vi "Remove Panel.vi"(0 "Shelf Number":string, 6 "connection information":path, 7 "System Num":u32=1 min=1 max=6) -> ()   [LabVIEW 2024]
uses:
  <vilib>/addons/database/Connection.llb/DB Tools Open Connec (Path).vi
  <vilib>/addons/database/Connection.llb/Conn Execute.vi
  <vilib>/addons/database/Recordset.llb/Rec Destroy - Connection.vi
  <vilib>/addons/database/_DB Variant To Data/Database Variant To Data.xnode
  <vilib>/addons/database/NI_Database_API.lvlib
panel:
  in  "Active Positions 2":string
  in  "Deselect All 2":bool
  in  "Select All 2":bool
  out "PreActive 2":string[](array[string])
  out "Rack 2":string
  out "Rack 1":string
  in  "13":bool
  in  "14":bool
  in  "15":bool
  in  "16":bool
  in  "21":bool
  in  "22":bool
  in  "23":bool
  in  "24":bool
  in  "29":bool
  in  "30":bool
  in  "31":bool
  in  "32":bool
  in  "10":bool
  in  "11":bool
  in  "12":bool
  in  "18":bool
  in  "19":bool
  in  "20":bool
  in  "26":bool
  in  "27":bool
  in  "28":bool
  in  "1":bool
  in  "2":bool
  in  "3":bool
  in  "4":bool
  in  "5":bool
  in  "6":bool
  in  "7":bool
  in  "8":bool
  in  "9":bool
  in  "17":bool
  in  "25":bool
  in  "Deselect All 1":bool
  out "PreActive 1":string[](array[string])
  out "System #":u32=1 min=1 max=6
  in  "Confirm":bool
  in  "Active Positions 1":string
  in  "13":bool
  in  "14":bool
  in  "15":bool
  in  "16":bool
  in  "21":bool
  in  "22":bool
  in  "23":bool
  in  "24":bool
  in  "29":bool
  in  "30":bool
  in  "31":bool
  in  "32":bool
  in  "10":bool
  in  "11":bool
  in  "12":bool
  in  "18":bool
  in  "19":bool
  in  "20":bool
  in  "26":bool
  in  "27":bool
  in  "28":bool
  in  "1":bool
  in  "2":bool
  in  "3":bool
  in  "4":bool
  in  "5":bool
  in  "6":bool
  in  "7":bool
  in  "8":bool
  in  "9":bool
  in  "17":bool
  in  "25":bool
  in  "Select All 1":bool
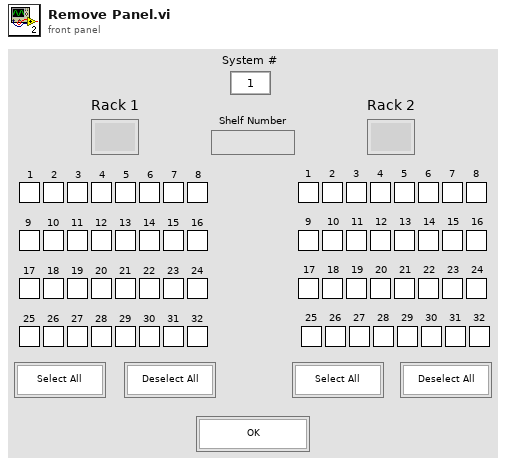
[diagram p1: front panel]
types:
  T1 = typedef "NI_Database_API.lvlib/Conn ObjectReference.ctl" = refnum<k1>
  T2 = typedef "NI_Database_API.lvlib/Rec ObjectReference.ctl" = refnum<k1>
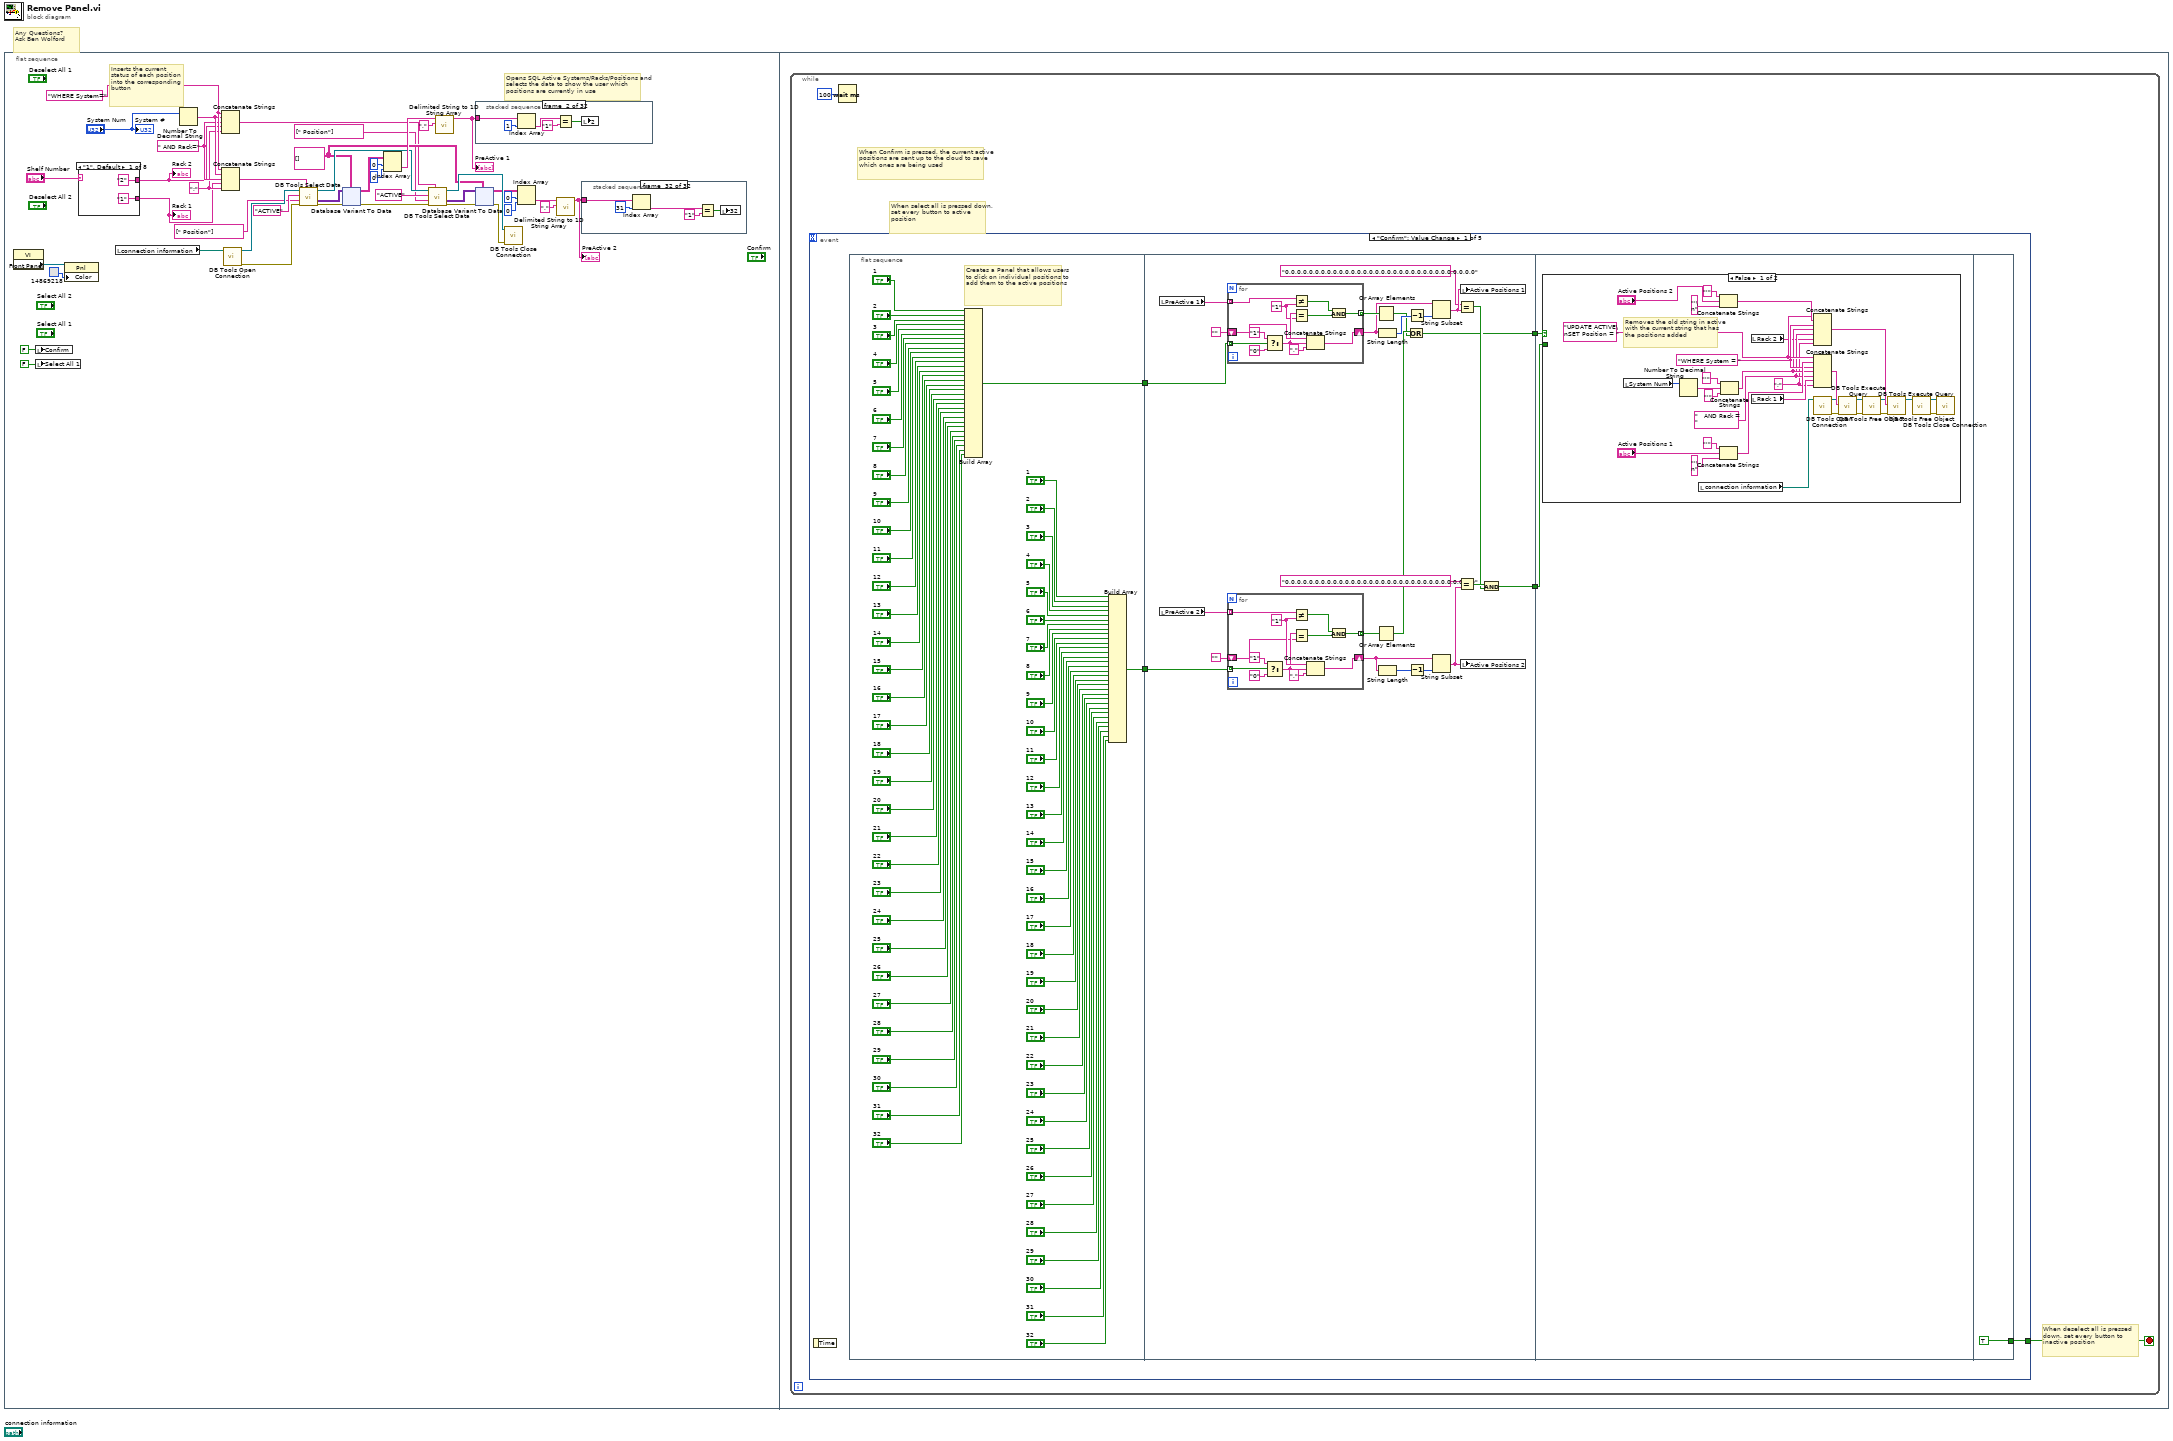
[diagram p0: block diagram]
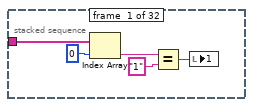
[diagram p2: hidden frame]
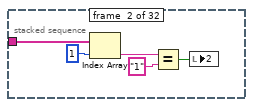
[diagram p3: hidden frame]
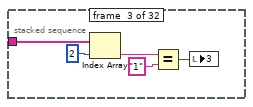
[diagram p4: hidden frame]
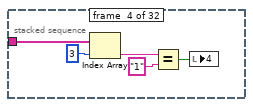
[diagram p5: hidden frame]
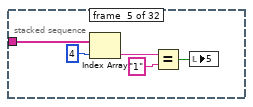
[diagram p6: hidden frame]
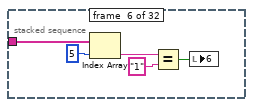
[diagram p7: hidden frame]
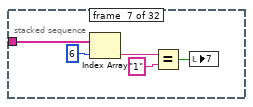
[diagram p8: hidden frame]
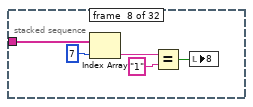
[diagram p9: hidden frame]
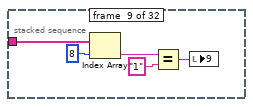
[diagram p10: hidden frame]
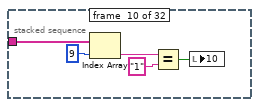
[diagram p11: hidden frame]
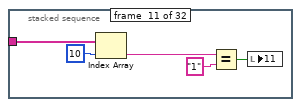
[diagram p12: hidden frame]
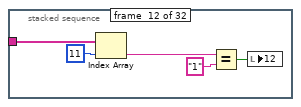
[diagram p13: hidden frame]
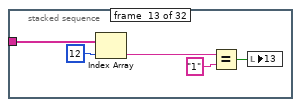
[diagram p14: hidden frame]
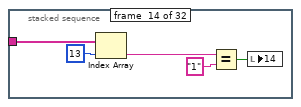
[diagram p15: hidden frame]
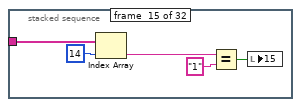
[diagram p16: hidden frame]
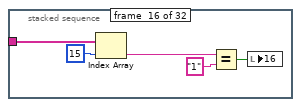
[diagram p17: hidden frame]
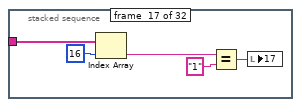
[diagram p18: hidden frame]
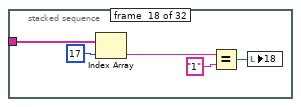
[diagram p19: hidden frame]
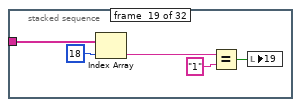
[diagram p20: hidden frame]
diagram:
  # "Any Questions? \nAsk Ben Wolford"
  n1 = flat-sequence {
    frame #0 {
      w5 = string[][] [] ("table")
      w29 = " AND Rack=" ("string")
      w28 = ";" ("string")
      w31 = "WHERE System=" ("SQL Query")
      # "Inserts the current status of each position into the corresponding button"
      # "Opens SQL Active Systems/Racks/Positions and selects the data to show the user which positions are currently in use"
      n2 = property class="VI"() -> ("Front Panel"=w34:refnum<vi>)  [unwired: 2 in, 2 out]
      n3 = local write "Confirm"(FALSE ("Confirm")) -> ()
      n4 = local write "Select All 1"(FALSE ("Select All")) -> ()
      n5 = property class="Pnl"(reference=w34, "Color"=u32 14869218) -> ()  [unwired: 1 in, 2 out]
      n6 = case shown="\"1\", Default" "Shelf Number" {
        tunnel: ["2" ("Rack 1") "4" ("Rack 1") "6" ("Rack 1") "8" ("Rack 1") "10" ("Rack 1") "12" ("Rack 1") "14" ("Rack 1") "16" ("Rack 1")] -> w26
        tunnel: ["1" ("Rack 1") "3" ("Rack 1") "5" ("Rack 1") "7" ("Rack 1") "9" ("Rack 1") "11" ("Rack 1") "13" ("Rack 1") "15" ("Rack 1")] -> w27
        frame "1", Default {
        }
        frame "2" {
        }
        frame "3" {
        }
        frame "4" {
        }
        frame "5" {
        }
        frame "6" {
        }
        frame "7" {
        }
        frame "8" {
        }
      }
      "Rack 1" <- w27
      "Rack 2" <- w26
      n7 = local read "connection information"() -> (w1:path)
      n8 = Number To Decimal String(number="System Num") -> (decimal integer string=w30:string)  [unwired: 1 in]
      n9 = Concatenate Strings(w31, w30, w29, w26, w28) -> (w4:string)
      n10 = Concatenate Strings(w31, w30, w29, w27, w28) -> (w8:string)
      n11 = call-poly <vilib>:"DB Tools Open Connection.vi"("connection information"=w1) -> ("error out"=w19:errorcluster, "connection reference"=w20:T1)  [unwired: 7 in]
      n12 = call <vilib>:"DB Tools Select Data.vi"("condition"=w8, "error in (no error)"=w19, "columns"=string[] [" Position"], "table"="ACTIVE", "connection reference"=w20) -> ("error out"=w14:errorcluster, "data"=w17:variant[][], "connection reference out"=w9:T1)  [unwired: 1 in]
      n13 = xnode "Database Variant To Data"("database variant"=w17, "error in (no error)"=w14, "type"=w5) -> ("data"=w7:string[][], "error out"=w13:errorcluster)
      n14 = Index Array(array=w7, index (row)=0, index (col)=0 ("disabled index (col)")) -> (element=w41:string)
      n15 = call <vilib>:"DB Tools Select Data.vi"("condition"=w4, "error in (no error)"=w13, "columns"=string[] [" Position"], "table"="ACTIVE", "connection reference"=w9) -> ("error out"=w12:errorcluster, "data"=w15:variant[][], "connection reference out"=w10:T1)  [unwired: 1 in]
      n16 = call <vilib>:"Delimited String to 1D String Array.vi"("delimiter"=",", "delimited string"=w41) -> ("string array"=w42:string[])  [unwired: 9 in]
      "PreActive 1" <- w42
      n17 = stacked-sequence {
        tunnel: w42 -> [w311 w313 w318 w323 w328 w333 w338 w343 w348 w353 w358 w363 w368 w373 w378 w383 w388 w393 w398 w403 w408 w413 w418 w423 w428 w433 w438 w443 w448 w453 w458 w463]
        frame #0 {
          n18 = Index Array(array=w311, index=0) -> (element=w309:string)
          n19 = Equal?(x=w309, y="1") -> (x = y?=w307:bool)
          n20 = local write "1"(w307) -> ()
        }
        frame #1 {
          n21 = Index Array(array=w313, index=1) -> (element=w315:string)
          n22 = Equal?(x=w315, y="1") -> (x = y?=w312:bool)
          n23 = local write "2"(w312) -> ()
        }
        frame #2 {
          n24 = Index Array(array=w318, index=2) -> (element=w320:string)
          n25 = Equal?(x=w320, y="1") -> (x = y?=w317:bool)
          n26 = local write "3"(w317) -> ()
        }
        frame #3 {
          n27 = Index Array(array=w323, index=3) -> (element=w325:string)
          n28 = Equal?(x=w325, y="1") -> (x = y?=w322:bool)
          n29 = local write "4"(w322) -> ()
        }
        frame #4 {
          n30 = Index Array(array=w328, index=4) -> (element=w330:string)
          n31 = Equal?(x=w330, y="1") -> (x = y?=w327:bool)
          n32 = local write "5"(w327) -> ()
        }
        frame #5 {
          n33 = Index Array(array=w333, index=5) -> (element=w335:string)
          n34 = Equal?(x=w335, y="1") -> (x = y?=w332:bool)
          n35 = local write "6"(w332) -> ()
        }
        frame #6 {
          n36 = Index Array(array=w338, index=6) -> (element=w340:string)
          n37 = Equal?(x=w340, y="1") -> (x = y?=w337:bool)
          n38 = local write "7"(w337) -> ()
        }
        frame #7 {
          n39 = Index Array(array=w343, index=7) -> (element=w345:string)
          n40 = Equal?(x=w345, y="1") -> (x = y?=w342:bool)
          n41 = local write "8"(w342) -> ()
        }
        frame #8 {
          n42 = Index Array(array=w348, index=8) -> (element=w350:string)
          n43 = Equal?(x=w350, y="1") -> (x = y?=w347:bool)
          n44 = local write "9"(w347) -> ()
        }
        frame #9 {
          n45 = Index Array(array=w353, index=9) -> (element=w355:string)
          n46 = Equal?(x=w355, y="1") -> (x = y?=w352:bool)
          n47 = local write "10"(w352) -> ()
        }
        frame #10 {
          n48 = Index Array(array=w358, index=10) -> (element=w360:string)
          n49 = Equal?(x=w360, y="1") -> (x = y?=w357:bool)
          n50 = local write "11"(w357) -> ()
        }
        frame #11 {
          n51 = Index Array(array=w363, index=11) -> (element=w365:string)
          n52 = Equal?(x=w365, y="1") -> (x = y?=w362:bool)
          n53 = local write "12"(w362) -> ()
        }
        frame #12 {
          n54 = Index Array(array=w368, index=12) -> (element=w370:string)
          n55 = Equal?(x=w370, y="1") -> (x = y?=w367:bool)
          n56 = local write "13"(w367) -> ()
        }
        frame #13 {
          n57 = Index Array(array=w373, index=13) -> (element=w375:string)
          n58 = Equal?(x=w375, y="1") -> (x = y?=w372:bool)
          n59 = local write "14"(w372) -> ()
        }
        frame #14 {
          n60 = Index Array(array=w378, index=14) -> (element=w380:string)
          n61 = Equal?(x=w380, y="1") -> (x = y?=w377:bool)
          n62 = local write "15"(w377) -> ()
        }
        frame #15 {
          n63 = Index Array(array=w383, index=15) -> (element=w385:string)
          n64 = Equal?(x=w385, y="1") -> (x = y?=w382:bool)
          n65 = local write "16"(w382) -> ()
        }
        frame #16 {
          n66 = Index Array(array=w388, index=16) -> (element=w390:string)
          n67 = Equal?(x=w390, y="1") -> (x = y?=w387:bool)
          n68 = local write "17"(w387) -> ()
        }
        frame #17 {
          n69 = Index Array(array=w393, index=17) -> (element=w395:string)
          n70 = Equal?(x=w395, y="1") -> (x = y?=w392:bool)
          n71 = local write "18"(w392) -> ()
        }
        frame #18 {
          n72 = Index Array(array=w398, index=18) -> (element=w400:string)
          n73 = Equal?(x=w400, y="1") -> (x = y?=w397:bool)
          n74 = local write "19"(w397) -> ()
        }
        frame #19 {
          n75 = Index Array(array=w403, index=19) -> (element=w405:string)
          n76 = Equal?(x=w405, y="1") -> (x = y?=w402:bool)
          n77 = local write "20"(w402) -> ()
        }
        frame #20 {
          n78 = Index Array(array=w408, index=20) -> (element=w410:string)
          n79 = Equal?(x=w410, y="1") -> (x = y?=w407:bool)
          n80 = local write "21"(w407) -> ()
        }
        frame #21 {
          n81 = Index Array(array=w413, index=21) -> (element=w415:string)
          n82 = Equal?(x=w415, y="1") -> (x = y?=w412:bool)
          n83 = local write "22"(w412) -> ()
        }
        frame #22 {
          n84 = Index Array(array=w418, index=22) -> (element=w420:string)
          n85 = Equal?(x=w420, y="1") -> (x = y?=w417:bool)
          n86 = local write "23"(w417) -> ()
        }
        frame #23 {
          n87 = Index Array(array=w423, index=23) -> (element=w425:string)
          n88 = Equal?(x=w425, y="1") -> (x = y?=w422:bool)
          n89 = local write "24"(w422) -> ()
        }
        frame #24 {
          n90 = Index Array(array=w428, index=24) -> (element=w430:string)
          n91 = Equal?(x=w430, y="1") -> (x = y?=w427:bool)
          n92 = local write "25"(w427) -> ()
        }
        frame #25 {
          n93 = Index Array(array=w433, index=25) -> (element=w435:string)
          n94 = Equal?(x=w435, y="1") -> (x = y?=w432:bool)
          n95 = local write "26"(w432) -> ()
        }
        frame #26 {
          n96 = Index Array(array=w438, index=26) -> (element=w440:string)
          n97 = Equal?(x=w440, y="1") -> (x = y?=w437:bool)
          n98 = local write "27"(w437) -> ()
        }
        frame #27 {
          n99 = Index Array(array=w443, index=27) -> (element=w445:string)
          n100 = Equal?(x=w445, y="1") -> (x = y?=w442:bool)
          n101 = local write "28"(w442) -> ()
        }
        frame #28 {
          n102 = Index Array(array=w448, index=28) -> (element=w450:string)
          n103 = Equal?(x=w450, y="1") -> (x = y?=w447:bool)
          n104 = local write "29"(w447) -> ()
        }
        frame #29 {
          n105 = Index Array(array=w453, index=29) -> (element=w455:string)
          n106 = Equal?(x=w455, y="1") -> (x = y?=w452:bool)
          n107 = local write "30"(w452) -> ()
        }
        frame #30 {
          n108 = Index Array(array=w458, index=30) -> (element=w460:string)
          n109 = Equal?(x=w460, y="1") -> (x = y?=w457:bool)
          n110 = local write "31"(w457) -> ()
        }
        frame #31 {
          n111 = Index Array(array=w463, index=31) -> (element=w465:string)
          n112 = Equal?(x=w465, y="1") -> (x = y?=w462:bool)
          n113 = local write "32"(w462) -> ()
        }
      }
      n114 = xnode "Database Variant To Data"("database variant"=w15, "error in (no error)"=w12, "type"=w5) -> ("data"=w6:string[][], "error out"=w11:errorcluster)
      n115 = call <vilib>:"DB Tools Close Connection.vi"("error in (no error)"=w11, "connection reference"=w10) -> ()  [unwired: 5 in, 1 out]
      n116 = Index Array(array=w6, index (row)=0, index (col)=0 ("disabled index (col)")) -> (element=w22:string)
      n117 = call <vilib>:"Delimited String to 1D String Array.vi"("delimiter"=",", "delimited string"=w22) -> ("string array"=w21:string[])  [unwired: 9 in]
      "PreActive 2" <- w21
      n118 = stacked-sequence {
        tunnel: w21 -> [w132 w137 w142 w147 w152 w157 w162 w167 w172 w177 w182 w187 w192 w197 w202 w207 w212 w217 w222 w227 w232 w237 w242 w247 w252 w257 w262 w267 w272 w277 w282 w287]
        frame #0 {
          n119 = Index Array(array=w132, index=0) -> (element=w134:string)
          n120 = Equal?(x=w134, y="1") -> (x = y?=w131:bool)
          n121 = local write "1"(w131) -> ()
        }
        frame #1 {
          n122 = Index Array(array=w137, index=1) -> (element=w139:string)
          n123 = Equal?(x=w139, y="1") -> (x = y?=w136:bool)
          n124 = local write "2"(w136) -> ()
        }
        frame #2 {
          n125 = Index Array(array=w142, index=2) -> (element=w144:string)
          n126 = Equal?(x=w144, y="1") -> (x = y?=w141:bool)
          n127 = local write "3"(w141) -> ()
        }
        frame #3 {
          n128 = Index Array(array=w147, index=3) -> (element=w149:string)
          n129 = Equal?(x=w149, y="1") -> (x = y?=w146:bool)
          n130 = local write "4"(w146) -> ()
        }
        frame #4 {
          n131 = Index Array(array=w152, index=4) -> (element=w154:string)
          n132 = Equal?(x=w154, y="1") -> (x = y?=w151:bool)
          n133 = local write "5"(w151) -> ()
        }
        frame #5 {
          n134 = Index Array(array=w157, index=5) -> (element=w159:string)
          n135 = Equal?(x=w159, y="1") -> (x = y?=w156:bool)
          n136 = local write "6"(w156) -> ()
        }
        frame #6 {
          n137 = Index Array(array=w162, index=6) -> (element=w164:string)
          n138 = Equal?(x=w164, y="1") -> (x = y?=w161:bool)
          n139 = local write "7"(w161) -> ()
        }
        frame #7 {
          n140 = Index Array(array=w167, index=7) -> (element=w169:string)
          n141 = Equal?(x=w169, y="1") -> (x = y?=w166:bool)
          n142 = local write "8"(w166) -> ()
        }
        frame #8 {
          n143 = Index Array(array=w172, index=8) -> (element=w174:string)
          n144 = Equal?(x=w174, y="1") -> (x = y?=w171:bool)
          n145 = local write "9"(w171) -> ()
        }
        frame #9 {
          n146 = Index Array(array=w177, index=9) -> (element=w179:string)
          n147 = Equal?(x=w179, y="1") -> (x = y?=w176:bool)
          n148 = local write "10"(w176) -> ()
        }
        frame #10 {
          n149 = Index Array(array=w182, index=10) -> (element=w184:string)
          n150 = Equal?(x=w184, y="1") -> (x = y?=w181:bool)
          n151 = local write "11"(w181) -> ()
        }
        frame #11 {
          n152 = Index Array(array=w187, index=11) -> (element=w189:string)
          n153 = Equal?(x=w189, y="1") -> (x = y?=w186:bool)
          n154 = local write "12"(w186) -> ()
        }
        frame #12 {
          n155 = Index Array(array=w192, index=12) -> (element=w194:string)
          n156 = Equal?(x=w194, y="1") -> (x = y?=w191:bool)
          n157 = local write "13"(w191) -> ()
        }
        frame #13 {
          n158 = Index Array(array=w197, index=13) -> (element=w199:string)
          n159 = Equal?(x=w199, y="1") -> (x = y?=w196:bool)
          n160 = local write "14"(w196) -> ()
        }
        frame #14 {
          n161 = Index Array(array=w202, index=14) -> (element=w204:string)
          n162 = Equal?(x=w204, y="1") -> (x = y?=w201:bool)
          n163 = local write "15"(w201) -> ()
        }
        frame #15 {
          n164 = Index Array(array=w207, index=15) -> (element=w209:string)
          n165 = Equal?(x=w209, y="1") -> (x = y?=w206:bool)
          n166 = local write "16"(w206) -> ()
        }
        frame #16 {
          n167 = Index Array(array=w212, index=16) -> (element=w214:string)
          n168 = Equal?(x=w214, y="1") -> (x = y?=w211:bool)
          n169 = local write "17"(w211) -> ()
        }
        frame #17 {
          n170 = Index Array(array=w217, index=17) -> (element=w219:string)
          n171 = Equal?(x=w219, y="1") -> (x = y?=w216:bool)
          n172 = local write "18"(w216) -> ()
        }
        frame #18 {
          n173 = Index Array(array=w222, index=18) -> (element=w224:string)
          n174 = Equal?(x=w224, y="1") -> (x = y?=w221:bool)
          n175 = local write "19"(w221) -> ()
        }
        frame #19 {
          n176 = Index Array(array=w227, index=19) -> (element=w229:string)
          n177 = Equal?(x=w229, y="1") -> (x = y?=w226:bool)
          n178 = local write "20"(w226) -> ()
        }
        frame #20 {
          n179 = Index Array(array=w232, index=20) -> (element=w234:string)
          n180 = Equal?(x=w234, y="1") -> (x = y?=w231:bool)
          n181 = local write "21"(w231) -> ()
        }
        frame #21 {
          n182 = Index Array(array=w237, index=21) -> (element=w239:string)
          n183 = Equal?(x=w239, y="1") -> (x = y?=w236:bool)
          n184 = local write "22"(w236) -> ()
        }
        frame #22 {
          n185 = Index Array(array=w242, index=22) -> (element=w244:string)
          n186 = Equal?(x=w244, y="1") -> (x = y?=w241:bool)
          n187 = local write "23"(w241) -> ()
        }
        frame #23 {
          n188 = Index Array(array=w247, index=23) -> (element=w249:string)
          n189 = Equal?(x=w249, y="1") -> (x = y?=w246:bool)
          n190 = local write "24"(w246) -> ()
        }
        frame #24 {
          n191 = Index Array(array=w252, index=24) -> (element=w254:string)
          n192 = Equal?(x=w254, y="1") -> (x = y?=w251:bool)
          n193 = local write "25"(w251) -> ()
        }
        frame #25 {
          n194 = Index Array(array=w257, index=25) -> (element=w259:string)
          n195 = Equal?(x=w259, y="1") -> (x = y?=w256:bool)
          n196 = local write "26"(w256) -> ()
        }
        frame #26 {
          n197 = Index Array(array=w262, index=26) -> (element=w264:string)
          n198 = Equal?(x=w264, y="1") -> (x = y?=w261:bool)
          n199 = local write "27"(w261) -> ()
        }
        frame #27 {
          n200 = Index Array(array=w267, index=27) -> (element=w269:string)
          n201 = Equal?(x=w269, y="1") -> (x = y?=w266:bool)
          n202 = local write "28"(w266) -> ()
        }
        frame #28 {
          n203 = Index Array(array=w272, index=28) -> (element=w274:string)
          n204 = Equal?(x=w274, y="1") -> (x = y?=w271:bool)
          n205 = local write "29"(w271) -> ()
        }
        frame #29 {
          n206 = Index Array(array=w277, index=29) -> (element=w279:string)
          n207 = Equal?(x=w279, y="1") -> (x = y?=w276:bool)
          n208 = local write "30"(w276) -> ()
        }
        frame #30 {
          n209 = Index Array(array=w282, index=30) -> (element=w284:string)
          n210 = Equal?(x=w284, y="1") -> (x = y?=w281:bool)
          n211 = local write "31"(w281) -> ()
        }
        frame #31 {
          n212 = Index Array(array=w287, index=31) -> (element=w289:string)
          n213 = Equal?(x=w289, y="1") -> (x = y?=w286:bool)
          n214 = local write "32"(w286) -> ()
        }
      }
      "System #" <- "System Num"
    }
    frame #1 {
      n215 = while {
        stop <- w467 stop-if-true
        # "When deselect all is pressed down, set every button to inactive position"
        # "When Confirm is pressed, the current active positions are sent up to the cloud to save which ones are being used"
        # "When select all is pressed down, set every button to active position"
        n216 = event shown="[0] \"Confirm\": Value Change" {
          selector: _ -> [_ _ _ _ _]
          dyn-events: _ -> [_ _ _ _ _]
          timeout: _ -> [_ _ _ _ _]
          tunnel: [w472 _ _ _ _] -> w467
          event "Confirm": Value Change {
            n217 = event-data() -> ()  [unwired: 1 in, 1 out]
            n218 = flat-sequence {
              tunnel: [w474] -> w473
              tunnel: [w475] -> w470
              tunnel: w473 -> [w561]
              tunnel: [w540] -> w471
              tunnel: w470 -> [w554]
              tunnel: [w543] -> w469
              tunnel: w471 -> [w589]
              tunnel: w469 -> [w588]
              tunnel: [TRUE] -> w472
              frame #0 {
                # "Creates a Panel that allows users to click on individual positions to add them to the active positions"
                n219 = Build Array("1", "2", "3", "4", "5", "6", "7", "8", "9", "10", "11", "12", "13", "14", "15", "16", "17", "18", "19", "20", "21", "22", "23", "24", "25", "26", "27", "28", "29", "30", "31", "32") -> (w474:bool[])
                n220 = Build Array("1", "2", "3", "4", "5", "6", "7", "8", "9", "10", "11", "12", "13", "14", "15", "16", "17", "18", "19", "20", "21", "22", "23", "24", "25", "26", "27", "28", "29", "30", "31", "32") -> (w475:bool[])
              }
              frame #1 {
                n221 = local read "PreActive 1"() -> (w557:string[])
                n222 = local read "PreActive 2"() -> (w553:string[])
                n223 = for {
                  tunnel: w561 -> [w582] mode=indexing
                  shift-right: [w586] -> w558
                  shift-left: "" -> [w587]
                  tunnel: w557 -> [w580] mode=indexing
                  tunnel: [w576] -> w559 mode=indexing
                  w579 = "1" ("y")
                  n224 = Select(t="1", s=w582, f="0") -> (s? t:f=w581:string)
                  n225 = Not Equal?(x=w580, y=w579) -> (x != y?=w577:bool)
                  n226 = Equal?(x=w581, y=w579) -> (x = y?=w578:bool)
                  n227 = Concatenate Strings(w587, w581, "," ("string")) -> (w586:string)
                  n228 = And(x=w577, y=w578) -> (x .and. y?=w576:bool)
                }
                n229 = for {
                  tunnel: w554 -> [w570] mode=indexing
                  shift-right: [w574] -> w548
                  shift-left: "" -> [w575]
                  tunnel: w553 -> [w568] mode=indexing
                  tunnel: [w564] -> w551 mode=indexing
                  w567 = "1" ("y")
                  n230 = Select(t="1", s=w570, f="0") -> (s? t:f=w569:string)
                  n231 = Not Equal?(x=w568, y=w567) -> (x != y?=w565:bool)
                  n232 = Equal?(x=w569, y=w567) -> (x = y?=w566:bool)
                  n233 = Concatenate Strings(w575, w569, "," ("string")) -> (w574:string)
                  n234 = And(x=w565, y=w566) -> (x .and. y?=w564:bool)
                }
                n235 = Or Array Elements(Boolean array=w559) -> (logical OR=w541:bool)
                n236 = Or Array Elements(Boolean array=w551) -> (logical OR=w542:bool)
                n237 = String Length(string=w558) -> (length=w562:i32)
                n238 = String Length(string=w548) -> (length=w549:i32)
                n239 = Or(x=w542, y=w541) -> (x .or. y?=w540:bool)
                n240 = Decrement(x=w562) -> (x-1=w563:i32)
                n241 = Decrement(x=w549) -> (x-1=w550:i32)
                n242 = String Subset(string=w558, length (rest)=w563) -> (substring=w556:string)  [unwired: 1 in]
                n243 = String Subset(string=w548, length (rest)=w550) -> (substring=w546:string)  [unwired: 1 in]
                n244 = Equal?(x="0,0,0,0,0,0,0,0,0,0,0,0,0,0,0,0,0,0,0,0,0,0,0,0,0,0,0,0,0,0,0,0", y=w556) -> (x = y?=w544:bool)
                n245 = Equal?(x="0,0,0,0,0,0,0,0,0,0,0,0,0,0,0,0,0,0,0,0,0,0,0,0,0,0,0,0,0,0,0,0", y=w546) -> (x = y?=w545:bool)
                n246 = local write "Active Positions 1"(w556) -> ()
                n247 = local write "Active Positions 2"(w546) -> ()
                n248 = And(x=w545, y=w544) -> (x .and. y?=w543:bool)
              }
              frame #2 {
                n249 = case shown="False" w589 {
                  tunnel: w588 -> [_ w622]
                  frame False {
                    w604 = "   AND Rack = " ("SQL Query")
                    w606 = "WHERE System = " ("SQL Query")
                    w602 = ";" ("string")
                    w607 = "UPDATE ACTIVE\nSET Position = " ("SQL Query")
                    # "Removes the old string in active with the current string that has the positions added"
                    n250 = local read "System Num"() -> (w620:u32)
                    n251 = Number To Decimal String(number=w620) -> (decimal integer string=w613:string)  [unwired: 1 in]
                    n252 = local read "connection information"() -> (w598:path)
                    n253 = Concatenate Strings("'" ("string"), "Active Positions 2", "'\n" ("string")) -> (w608:string)
                    n254 = Concatenate Strings("'" ("string"), "Active Positions 1", "'\n" ("string")) -> (w616:string)
                    n255 = Concatenate Strings("'" ("string"), w613, "'" ("string")) -> (w605:string)
                    n256 = local read "Rack 2"() -> (w603:string)
                    n257 = local read "Rack 1"() -> (w612:string)
                    n258 = Concatenate Strings(w607, w608, w606, w605, w604, w603, w602) -> (w600:string)
                    n259 = Concatenate Strings(w607, w616, w606, w605, w604, w612, w602) -> (w601:string)
                    n260 = call-poly <vilib>:"DB Tools Open Connection.vi"("connection information"=w598) -> ("error out"=w599:errorcluster, "connection reference"=w595:T1)  [unwired: 7 in]
                    n261 = call-poly <vilib>:"DB Tools Execute Query.vi"("error in (no error)"=w599, "SQL query"=w601, "connection reference"=w595) -> ("error out"=w597:errorcluster, "recordset reference"=w596:T2)  [unwired: 5 in]
                    n262 = call-poly <vilib>:"DB Tools Free Object.vi"("error in (no error)"=w597, "recordset reference"=w596) -> ("error out"=w590:errorcluster, "connection reference"=w594:T1)  [unwired: 8 in]
                    n263 = call-poly <vilib>:"DB Tools Execute Query.vi"("error in (no error)"=w590, "SQL query"=w600, "connection reference"=w594) -> ("recordset reference"=w593:T2)  [unwired: 5 in, 1 out]
                    n264 = call-poly <vilib>:"DB Tools Free Object.vi"("recordset reference"=w593) -> ("error out"=w591:errorcluster, "connection reference"=w592:T1)  [unwired: 9 in]
                    n265 = call <vilib>:"DB Tools Close Connection.vi"("error in (no error)"=w591, "connection reference"=w592) -> ()  [unwired: 5 in, 1 out]
                  }
                  frame True {
                    n266 = Not(x=w622) -> (.not. x?=w621:bool)
                    n267 = call "Display Message to User"("Enable"=w621) -> ()  [unwired: 9 in, 2 out]
                  }
                }
              }
              frame #3 {
              }
            }
          }
          event "Select All 1": Value Change {
            # "Turns all of the buttons/positions to true"
            n268 = event-data() -> ()  [unwired: 1 in, 3 out]
            n269 = stacked-sequence {
              frame #0 {
                n270 = local write "1"(TRUE) -> ()
              }
              frame #1 {
                n271 = local write "2"(TRUE) -> ()
              }
              frame #2 {
                n272 = local write "3"(TRUE) -> ()
              }
              frame #3 {
                n273 = local write "4"(TRUE) -> ()
              }
              frame #4 {
                n274 = local write "5"(TRUE) -> ()
              }
              frame #5 {
                n275 = local write "6"(TRUE) -> ()
              }
              frame #6 {
                n276 = local write "7"(TRUE) -> ()
              }
              frame #7 {
                n277 = local write "8"(TRUE) -> ()
              }
              frame #8 {
                n278 = local write "9"(TRUE) -> ()
              }
              frame #9 {
                n279 = local write "10"(TRUE) -> ()
              }
              frame #10 {
                n280 = local write "11"(TRUE) -> ()
              }
              frame #11 {
                n281 = local write "12"(TRUE) -> ()
              }
              frame #12 {
                n282 = local write "13"(TRUE) -> ()
              }
              frame #13 {
                n283 = local write "14"(TRUE) -> ()
              }
              frame #14 {
                n284 = local write "15"(TRUE) -> ()
              }
              frame #15 {
                n285 = local write "16"(TRUE) -> ()
              }
              frame #16 {
                n286 = local write "17"(TRUE) -> ()
              }
              frame #17 {
                n287 = local write "18"(TRUE) -> ()
              }
              frame #18 {
                n288 = local write "19"(TRUE) -> ()
              }
              frame #19 {
                n289 = local write "20"(TRUE) -> ()
              }
              frame #20 {
                n290 = local write "21"(TRUE) -> ()
              }
              frame #21 {
                n291 = local write "22"(TRUE) -> ()
              }
              frame #22 {
                n292 = local write "23"(TRUE) -> ()
              }
              frame #23 {
                n293 = local write "24"(TRUE) -> ()
              }
              frame #24 {
                n294 = local write "25"(TRUE) -> ()
              }
              frame #25 {
                n295 = local write "26"(TRUE) -> ()
              }
              frame #26 {
                n296 = local write "27"(TRUE) -> ()
              }
              frame #27 {
                n297 = local write "28"(TRUE) -> ()
              }
              frame #28 {
                n298 = local write "29"(TRUE) -> ()
              }
              frame #29 {
                n299 = local write "30"(TRUE) -> ()
              }
              frame #30 {
                n300 = local write "31"(TRUE) -> ()
              }
              frame #31 {
                n301 = local write "32"(TRUE) -> ()
              }
            }
          }
          event "Select All 2": Value Change {
            # "Turns all of the buttons/positions to true"
            n302 = event-data() -> ()  [unwired: 1 in, 3 out]
            n303 = stacked-sequence {
              frame #0 {
                n304 = local write "1"(TRUE) -> ()
              }
              frame #1 {
                n305 = local write "2"(TRUE) -> ()
              }
              frame #2 {
                n306 = local write "3"(TRUE) -> ()
              }
              frame #3 {
                n307 = local write "4"(TRUE) -> ()
              }
              frame #4 {
                n308 = local write "5"(TRUE) -> ()
              }
              frame #5 {
                n309 = local write "6"(TRUE) -> ()
              }
              frame #6 {
                n310 = local write "7"(TRUE) -> ()
              }
              frame #7 {
                n311 = local write "8"(TRUE) -> ()
              }
              frame #8 {
                n312 = local write "9"(TRUE) -> ()
              }
              frame #9 {
                n313 = local write "10"(TRUE) -> ()
              }
              frame #10 {
                n314 = local write "11"(TRUE) -> ()
              }
              frame #11 {
                n315 = local write "12"(TRUE) -> ()
              }
              frame #12 {
                n316 = local write "13"(TRUE) -> ()
              }
              frame #13 {
                n317 = local write "14"(TRUE) -> ()
              }
              frame #14 {
                n318 = local write "15"(TRUE) -> ()
              }
              frame #15 {
                n319 = local write "16"(TRUE) -> ()
              }
              frame #16 {
                n320 = local write "17"(TRUE) -> ()
              }
              frame #17 {
                n321 = local write "18"(TRUE) -> ()
              }
              frame #18 {
                n322 = local write "19"(TRUE) -> ()
              }
              frame #19 {
                n323 = local write "20"(TRUE) -> ()
              }
              frame #20 {
                n324 = local write "21"(TRUE) -> ()
              }
              frame #21 {
                n325 = local write "22"(TRUE) -> ()
              }
              frame #22 {
                n326 = local write "23"(TRUE) -> ()
              }
              frame #23 {
                n327 = local write "24"(TRUE) -> ()
              }
              frame #24 {
                n328 = local write "25"(TRUE) -> ()
              }
              frame #25 {
                n329 = local write "26"(TRUE) -> ()
              }
              frame #26 {
                n330 = local write "27"(TRUE) -> ()
              }
              frame #27 {
                n331 = local write "28"(TRUE) -> ()
              }
              frame #28 {
                n332 = local write "29"(TRUE) -> ()
              }
              frame #29 {
                n333 = local write "30"(TRUE) -> ()
              }
              frame #30 {
                n334 = local write "31"(TRUE) -> ()
              }
              frame #31 {
                n335 = local write "32"(TRUE) -> ()
              }
            }
          }
          event "Deselect All 1": Value Change {
            # "Turns all of the buttons/positions to false"
            n336 = event-data() -> ()  [unwired: 1 in, 3 out]
            n337 = stacked-sequence {
              frame #0 {
                n338 = local write "1"(FALSE) -> ()
              }
              frame #1 {
                n339 = local write "2"(FALSE) -> ()
              }
              frame #2 {
                n340 = local write "3"(FALSE) -> ()
              }
              frame #3 {
                n341 = local write "4"(FALSE) -> ()
              }
              frame #4 {
                n342 = local write "5"(FALSE) -> ()
              }
              frame #5 {
                n343 = local write "6"(FALSE) -> ()
              }
              frame #6 {
                n344 = local write "7"(FALSE) -> ()
              }
              frame #7 {
                n345 = local write "8"(FALSE) -> ()
              }
              frame #8 {
                n346 = local write "9"(FALSE) -> ()
              }
              frame #9 {
                n347 = local write "10"(FALSE) -> ()
              }
              frame #10 {
                n348 = local write "11"(FALSE) -> ()
              }
              frame #11 {
                n349 = local write "12"(FALSE) -> ()
              }
              frame #12 {
                n350 = local write "13"(FALSE) -> ()
              }
              frame #13 {
                n351 = local write "14"(FALSE) -> ()
              }
              frame #14 {
                n352 = local write "15"(FALSE) -> ()
              }
              frame #15 {
                n353 = local write "16"(FALSE) -> ()
              }
              frame #16 {
                n354 = local write "17"(FALSE) -> ()
              }
              frame #17 {
                n355 = local write "18"(FALSE) -> ()
              }
              frame #18 {
                n356 = local write "19"(FALSE) -> ()
              }
              frame #19 {
                n357 = local write "20"(FALSE) -> ()
              }
              frame #20 {
                n358 = local write "21"(FALSE) -> ()
              }
              frame #21 {
                n359 = local write "22"(FALSE) -> ()
              }
              frame #22 {
                n360 = local write "23"(FALSE) -> ()
              }
              frame #23 {
                n361 = local write "24"(FALSE) -> ()
              }
              frame #24 {
                n362 = local write "25"(FALSE) -> ()
              }
              frame #25 {
                n363 = local write "26"(FALSE) -> ()
              }
              frame #26 {
                n364 = local write "27"(FALSE) -> ()
              }
              frame #27 {
                n365 = local write "28"(FALSE) -> ()
              }
              frame #28 {
                n366 = local write "29"(FALSE) -> ()
              }
              frame #29 {
                n367 = local write "30"(FALSE) -> ()
              }
              frame #30 {
                n368 = local write "31"(FALSE) -> ()
              }
              frame #31 {
                n369 = local write "32"(FALSE) -> ()
              }
            }
          }
          event "Deselect All 2": Value Change {
            # "Turns all of the buttons/positions to false"
            n370 = event-data() -> ()  [unwired: 1 in, 3 out]
            n371 = stacked-sequence {
              frame #0 {
                n372 = local write "1"(FALSE) -> ()
              }
              frame #1 {
                n373 = local write "2"(FALSE) -> ()
              }
              frame #2 {
                n374 = local write "3"(FALSE) -> ()
              }
              frame #3 {
                n375 = local write "4"(FALSE) -> ()
              }
              frame #4 {
                n376 = local write "5"(FALSE) -> ()
              }
              frame #5 {
                n377 = local write "6"(FALSE) -> ()
              }
              frame #6 {
                n378 = local write "7"(FALSE) -> ()
              }
              frame #7 {
                n379 = local write "8"(FALSE) -> ()
              }
              frame #8 {
                n380 = local write "9"(FALSE) -> ()
              }
              frame #9 {
                n381 = local write "10"(FALSE) -> ()
              }
              frame #10 {
                n382 = local write "11"(FALSE) -> ()
              }
              frame #11 {
                n383 = local write "12"(FALSE) -> ()
              }
              frame #12 {
                n384 = local write "13"(FALSE) -> ()
              }
              frame #13 {
                n385 = local write "14"(FALSE) -> ()
              }
              frame #14 {
                n386 = local write "15"(FALSE) -> ()
              }
              frame #15 {
                n387 = local write "16"(FALSE) -> ()
              }
              frame #16 {
                n388 = local write "17"(FALSE) -> ()
              }
              frame #17 {
                n389 = local write "18"(FALSE) -> ()
              }
              frame #18 {
                n390 = local write "19"(FALSE) -> ()
              }
              frame #19 {
                n391 = local write "20"(FALSE) -> ()
              }
              frame #20 {
                n392 = local write "21"(FALSE) -> ()
              }
              frame #21 {
                n393 = local write "22"(FALSE) -> ()
              }
              frame #22 {
                n394 = local write "23"(FALSE) -> ()
              }
              frame #23 {
                n395 = local write "24"(FALSE) -> ()
              }
              frame #24 {
                n396 = local write "25"(FALSE) -> ()
              }
              frame #25 {
                n397 = local write "26"(FALSE) -> ()
              }
              frame #26 {
                n398 = local write "27"(FALSE) -> ()
              }
              frame #27 {
                n399 = local write "28"(FALSE) -> ()
              }
              frame #28 {
                n400 = local write "29"(FALSE) -> ()
              }
              frame #29 {
                n401 = local write "30"(FALSE) -> ()
              }
              frame #30 {
                n402 = local write "31"(FALSE) -> ()
              }
              frame #31 {
                n403 = local write "32"(FALSE) -> ()
              }
            }
          }
        }
        n404 = Wait (ms)(milliseconds to wait=u32 100) -> ()  [unwired: 1 out]
      }
    }
  }
